vi "init.vi"(8 "error in (no error)":errorcluster, 11 "DualActingPneumaticCylinder_Lateral in":refnum<class "DualActingPneumaticCylinder_Lateral.lvclass">) -> (0 "error out":errorcluster, 3 "DualActingPneumaticCylinder_Lateral out":refnum<class "DualActingPneumaticCylinder_Lateral.lvclass">)   [LabVIEW 2013, in "DualActingPneumaticCylinder_Lateral.lvclass"]
uses:
  DualActingPneumaticCylinder_Lateral.lvclass
  PressureTransducerCompensator_Lateral/PressureTransducerCompensator_Lateral.lvclass
  FlowControlValveCompensator_Lateral/FlowControlValveCompensator_Lateral.lvclass
  DualActingPneumaticCylinder/DualActingPneumaticCylinder.lvclass/DualActingPneumaticCylinder.ctl
  PressureTransducerCompensator/PressureTransducerCompensator.lvclass
  FlowControlValveCompensator/FlowControlValveCompensator.lvclass
  DualActingPneumaticCylinder/DualActingPneumaticCylinder.lvclass
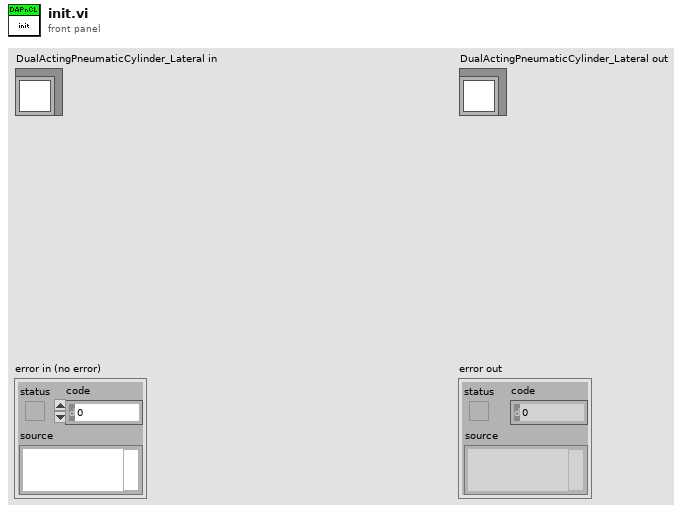
[diagram p1: front panel]
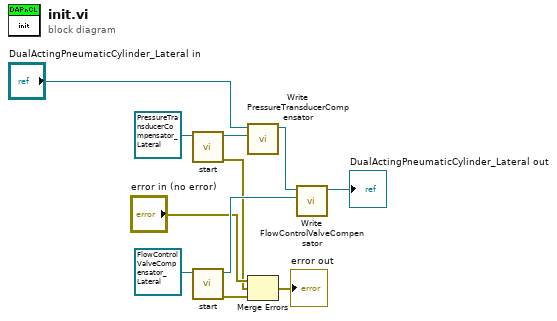
[diagram p0: block diagram]
diagram:
  n1 = call "start.vi"("PressureTransducerCompensator in"=refnum<class "PressureTransducerCompensator_Lateral.lvclass"> refnum ("PressureTransducerCompensator_Lateral.lvclass")) -> ("error out"=w2:errorcluster, "PressureTransducerCompensator out"=w9:refnum<class "PressureTransducerCompensator_Lateral.lvclass">)  [unwired: 9 in]
  n2 = call "start.vi"("FlowControlValveCompensator in"=refnum<class "FlowControlValveCompensator_Lateral.lvclass"> refnum ("FlowControlValveCompensator_Lateral.lvclass")) -> ("error out"=w3:errorcluster, "FlowControlValveCompensator out"=w5:refnum<class "FlowControlValveCompensator_Lateral.lvclass">)  [unwired: 9 in]
  n3 = call "Write PressureTransducerCompensator.vi"("PressureTransducerCompensator.lvclass"=w9, "DualActingPneumaticCylinder in"="DualActingPneumaticCylinder_Lateral in") -> ("DualActingPneumaticCylinder out"=w7:refnum<class "DualActingPneumaticCylinder_Lateral.lvclass">)  [unwired: 9 in]
  n4 = Merge Errors("error in (no error)", w2, w3) -> (→"error out":errorcluster)
  n5 = call "Write FlowControlValveCompensator.vi"("FlowControlValveCompensator.lvclass"=w5, "DualActingPneumaticCylinder in"=w7) -> ("DualActingPneumaticCylinder out"=→"DualActingPneumaticCylinder_Lateral out":refnum<class "DualActingPneumaticCylinder_Lateral.lvclass">)  [unwired: 9 in]
